vi "Main.vi"() -> ()   [LabVIEW 2016]
uses:
  Code/MainFGV/MainFGV_mods.ctl
  <vilib>/DAQmx/read.llb/DAQmx Read (Analog 2D DBL NChan NSamp).vi
  <vilib>/DAQmx/miscellaneous.llb/DAQmx Fill In Error Info.vi
panel:
  out "error out":errorcluster
  in  "simulation":bool
  in  "Log":string
  in  "tab":enum32{"Extensômetros", "Molinetes"}(tab)
  in  "stop":bool
  in  "Iniciar ensaio":bool
  in  "TestName":string caption="Nome do ensaio"
  in  "config":bool
  in  "TesrtDir":path caption="Diretório do ensaio"
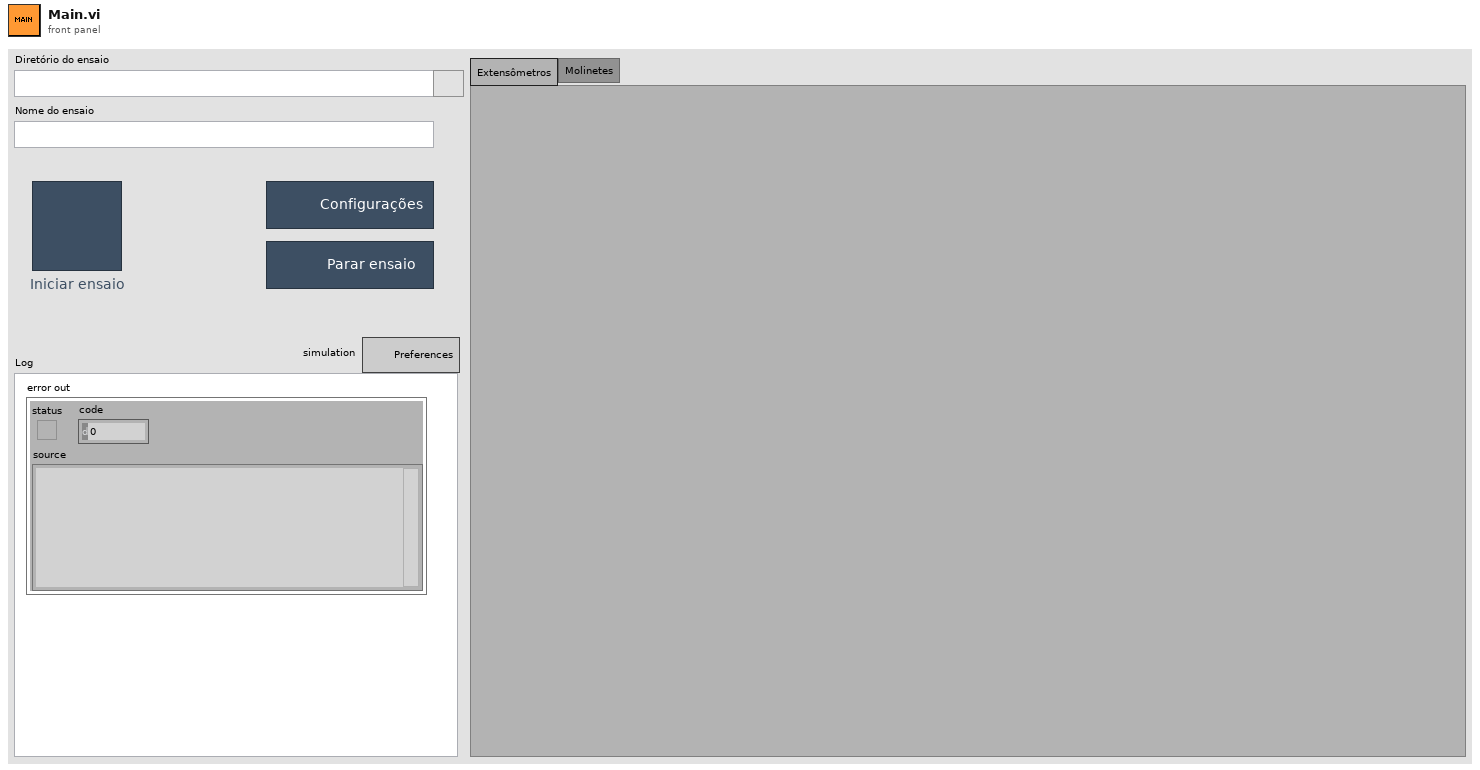
[diagram p1: front panel]
types:
  T1 = typedef "MainFGV_mods.ctl" = enum16{"Init", "Config", "CreateTask", "Register", "Start", "Record", "End"}
  T2 = cluster{"simulation":bool, "TesrtDir":path, "TestName":string}
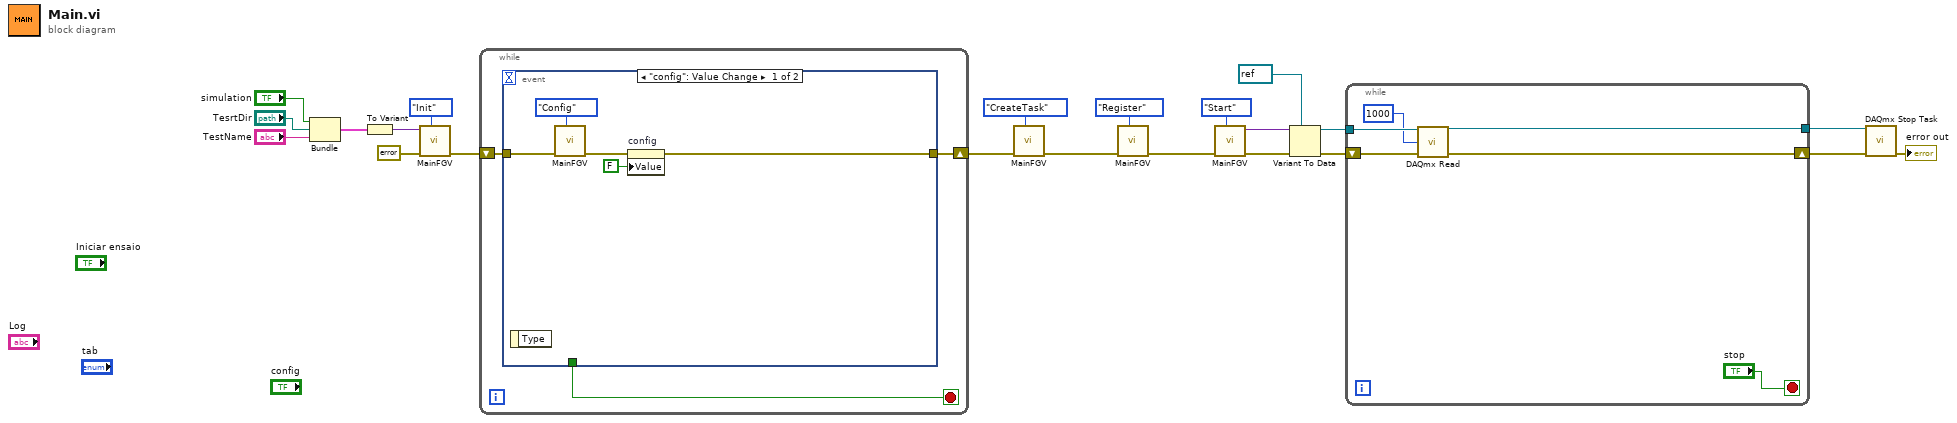
[diagram p0: block diagram]
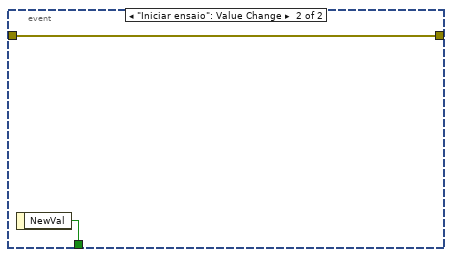
[diagram p2: hidden frame]
diagram:
  n1 = Bundle("simulation"="simulation", "TesrtDir"="TesrtDir", "TestName"="TestName") -> (w19:T2)  [unwired: 1 in]
  n2 = To Variant(anything=w19) -> (Variant=w18:variant)
  n3 = call "MainFGV.vi"("FGV_mods"=MainFGV_mods."Init", "Error In"=errorcluster {"status"=FALSE, "code"=0, "source"=""}, "DataIn"=w18) -> ("Error Out"=w16:errorcluster)  [unwired: 7 in, 1 out]
  n4 = while {
    shift-right: [w24] -> w13
    shift-left: w16 -> [w25]
    stop <- w23 stop-if-true
    n5 = event shown="[0] \"config\": Value Change" {
      selector: _ -> [_ _]
      dyn-events: _ -> [_ _]
      timeout: _ -> [_ _]
      tunnel: w25 -> [w29 w31]
      tunnel: [w27 w31] -> w24
      tunnel: [_ w32] -> w23
      event "config": Value Change {
        n6 = event-data() -> ()  [unwired: 1 in, 1 out]
        n7 = call "MainFGV.vi"("FGV_mods"=MainFGV_mods."Config", "Error In"=w29) -> ("Error Out"=w28:errorcluster)  [unwired: 8 in, 1 out]
        n8 = property on="config" class="Bool (strict)"(error in=w28, "Value"=FALSE ("config")) -> (error out=w27:errorcluster)  [unwired: 1 in, 1 out]
      }
      event "Iniciar ensaio": Value Change {
        n9 = event-data() -> ("NewVal"=w32:bool)  [unwired: 1 in]
      }
    }
  }
  n10 = call "MainFGV.vi"("FGV_mods"=MainFGV_mods."CreateTask", "Error In"=w13) -> ("Error Out"=w11:errorcluster)  [unwired: 8 in, 1 out]
  n11 = call "MainFGV.vi"("FGV_mods"=MainFGV_mods."Register", "Error In"=w11) -> ("Error Out"=w9:errorcluster)  [unwired: 8 in, 1 out]
  n12 = call "MainFGV.vi"("FGV_mods"=MainFGV_mods."Start", "Error In"=w9) -> ("Error Out"=w8:errorcluster, "DataOut"=w7:variant)  [unwired: 8 in]
  n13 = Variant To Data(error in=w8, type=refnum<k21> refnum ("task out"), Variant=w7) -> (data=w5:refnum<k21>, error out=w4:errorcluster)
  n14 = while {
    tunnel: w5 -> [w38]
    shift-right: [w36] -> w3
    shift-left: w4 -> [w37]
    tunnel: [w35] -> w2
    stop <- "stop" stop-if-true
    n15 = call-poly <vilib>:"DAQmx Read.vi"("task/channels in"=w38, "number of samples per channel"=1000, "error in"=w37) -> ("task out"=w35:refnum<k21>, "error out"=w36:errorcluster)  [unwired: 10 in, 1 out]
  }
  n16 = call <vilib>:"DAQmx Stop Task.vi"("task/channels in"=w2, "error in"=w3) -> ("error out"=→"error out":errorcluster)  [unwired: 12 in, 1 out]
